vi "bp debug.vi"() -> ()   [LabVIEW 2021]
uses:
  TypeDefs/Write Configuration.ctl
  TypeDefs/Read Configuration.ctl
  TypeDefs/Read Position.ctl
  b69df9f4-e5c4-46b9-b803-5522842ebdb0.vi
  c07a2b01-f723-416f-a3fc-56ab7bb24a60.vi
  4c0453df-4ba6-4fa7-9bdd-2c7ed909ac70.vi
  8cb2bc32-5875-4f0f-96cf-53a1e95d2331.vi
  b69df9f4-e5c4-46b9-b803-5522842ebdb0.vi/49b3dd2d-4579-4089-b72e-3f0875c862f2.vi
  SubVIs/Check Error.vi
  SubVIs/Add CIPC Error.vi
  SubVIs/Get dll Path.vi
  c07a2b01-f723-416f-a3fc-56ab7bb24a60.vi/ad4ed45e-f2aa-403d-a38b-be52afbcecdf.vi
  SubVIs/Notify Of New Write.vi
  8cb2bc32-5875-4f0f-96cf-53a1e95d2331.vi/ad4ed45e-f2aa-403d-a38b-be52afbcecdf.vi
  <vilib>/CIF Foundation/CIF Utilities/Errors/Append Error Location.vi
  SubVIs/Wait For N Elements Available.vi
  <vilib>/Utility/error.llb/Trim Whitespace.vi
  <vilib>/string/Create NI GUID.vi
  SubVIs/Get Element Description Variant.vi
  <vilib>/Utility/error.llb/Error Cluster From Error Code.vi
  SubVIs/Get Element Info Variant.vi
  CIF_NI_CIPC.lvlib
panel:
  out "Element Read Position 2":u32
  out "Index 2":u32
  out "Element Read Position":u32
  out "Index":u32
  out "Success 2":bool
  out "Success":bool
  out "Data out":i32
  out "error out":errorcluster
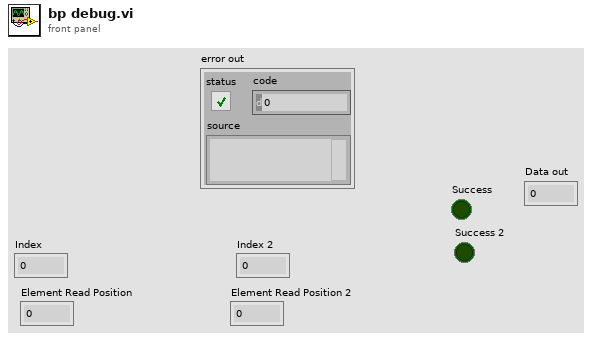
[diagram p1: front panel]
types:
  T1 = typedef "CIF_NI_CIPC.lvlib/Read Position.ctl" = enum16{"Next", "Newest", "Oldest", "Next Available", "Absolute"}
  T2 = typedef "CIF_NI_CIPC.lvlib/Read Configuration.ctl" = cluster{"Read Position":T1, "Element Offset":i32, "Prepend Array Size":bool, "Get Read Position":bool}
  T3 = typedef "CIF_NI_CIPC.lvlib/Write Configuration.ctl" = cluster{"Prepend Array Size":bool, "Get Write Position":bool, "Notify Readers":bool}
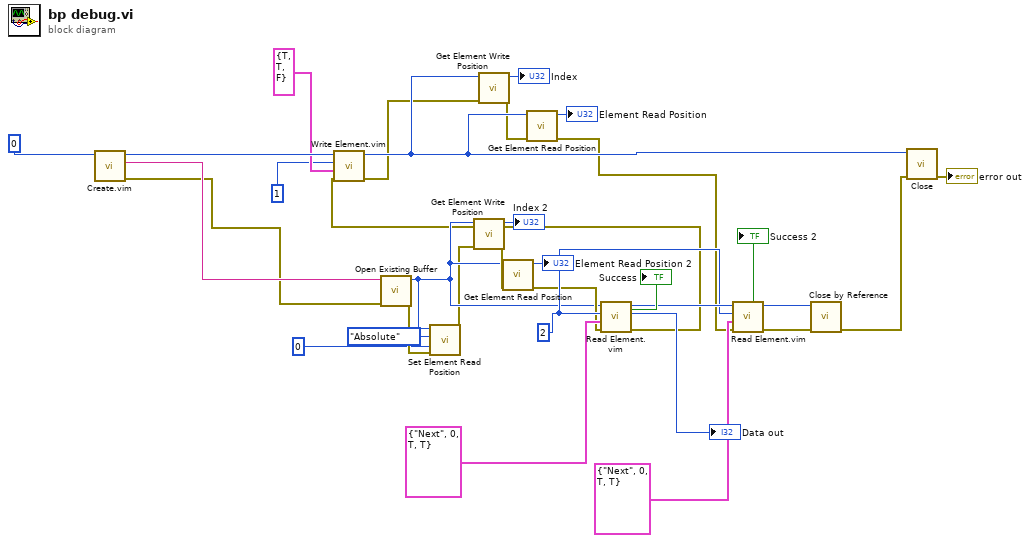
[diagram p0: block diagram]
diagram:
  w22 = 2
  n1 = call "Create.vim"("Data Type"=0) -> ("error out"=w3:errorcluster, "Name out"=w32:string, "CIPC Reference"=w6:u64)  [unwired: 7 in, 1 out]
  n2 = call "Open Existing Buffer.vi"("error in (no error)"=w3, "buffer_name"=w32) -> ("error out"=w10:errorcluster, "CIPC Reference"=w11:u64)  [unwired: 8 in]
  n3 = call "Set Element Read Position.vi"("error in (no error)"=w10, "Element Index Offset"=0, "Read Position"=Read_Position."Absolute", "CIPC Reference"=w11) -> ("error out"=w7:errorcluster)  [unwired: 7 in]
  n4 = call "Get Element Write Position.vi"("error in (no error)"=w7, "CIPC Reference"=w11) -> ("error out"=w20:errorcluster, "Index"=→"Index 2":u32)  [unwired: 8 in]
  n5 = call "Get Element Read Position.vi"("error in (no error)"=w20, "CIPC Reference"=w11) -> ("error out"=w19:errorcluster, "Element Read Position"=→"Element Read Position 2":u32)  [unwired: 8 in]
  n6 = call "Read Element.vim"("error in"=w19, "Read Configuration"=T2 {"Read Position"=enum."Next", "Element Offset"=0, "Prepend Array Size"=TRUE, "Get Read Position"=TRUE}, "Data in"=w22, "CIPC Reference in"=w11) -> ("error out"=w2:errorcluster, "Data out"=→"Data out":i32, "CIPC Reference out"=w26:u64, "Success"=→"Success":bool)  [unwired: 3 in, 1 out]
  n7 = call "Write Element.vim"("error in (no error)"=w2, "Write Configuration"=T3 {"Prepend Array Size"=TRUE, "Get Write Position"=TRUE, "Notify Readers"=FALSE}, "Data in"=1, "CIPC Reference in"=w6) -> ("error out"=w12:errorcluster, "CIPC Reference out"=w18:u64)  [unwired: 4 in, 2 out]
  n8 = call "Get Element Write Position.vi"("error in (no error)"=w12, "CIPC Reference"=w18) -> ("error out"=w17:errorcluster, "Index"=→"Index":u32)  [unwired: 8 in]
  n9 = call "Get Element Read Position.vi"("error in (no error)"=w17, "CIPC Reference"=w18) -> ("error out"=w1:errorcluster, "Element Read Position"=→"Element Read Position":u32)  [unwired: 8 in]
  n10 = call "Read Element.vim"("error in"=w1, "Read Configuration"=T2 {"Read Position"=enum."Next", "Element Offset"=0, "Prepend Array Size"=TRUE, "Get Read Position"=TRUE}, "Data in"=w22, "CIPC Reference in"=w26) -> ("error out"=w25:errorcluster, "CIPC Reference out"=w24:u64, "Success"=→"Success 2":bool)  [unwired: 3 in, 2 out]
  n11 = call "Close by Reference.vi"("error in (no error)"=w25, "CIPC Reference"=w24) -> ("error out"=w31:errorcluster)  [unwired: 9 in]
  n12 = call "Close.vi"("error in (no error)"=w31, "CIPC Reference"=w18) -> ("error out"=→"error out":errorcluster)  [unwired: 9 in]
